vi "createSection.vi"(8 "error in (no error)":errorcluster, 10 "Style":refnum<class "Style.lvclass">, 11 "Paragraph in":refnum<k24>) -> (0 "error out":errorcluster, 2 "Section out":refnum<k24>, 3 "Paragraph out":refnum<k24>)   [LabVIEW 2017, in "LabVIEW NPOI.lvlib" / "xwpfWriter.lvclass"]
uses:
  xwpfWriter.lvclass
  Styles/Style/Style.lvclass
  C:/Users/Neo/Desktop/Dev_Tools_BR/LabVIEW_NPOI/lib/NPOI 2.1.1/NPOI.OOXML.dll
  lib/NPOI 2.1.1/NPOI.OOXML.dll
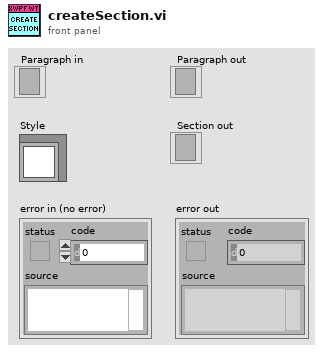
[diagram p1: front panel]
types:
  T1 = typedef "Styles.lvlib/Alignment--ring.ctl" = i32
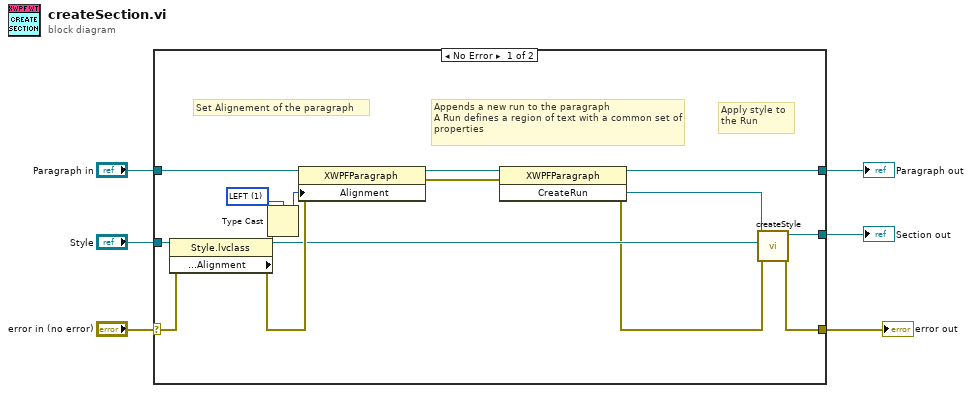
[diagram p0: block diagram]
diagram:
  n1 = case shown="No Error" "error in (no error)" {
    selector: "error in (no error)" -> [w17 w23]
    tunnel: [w12 w23] -> w5
    tunnel: "Style" -> [w21 _]
    tunnel: "Paragraph in" -> [w16 w22]
    tunnel: [w11 w22] -> w2
    tunnel: [w10 _] -> w1
    frame No Error {
      w9 = 1 items=["LEFT"=1, "CENTER"=2, "RIGHT"=3, "BOTH"=4, "MEDIUM_KASHIDA"=5, "DISTRIBUTE"=6, "NUM_TAB"=7, "HIGH_KASHIDA"=8, "LOW_KASHIDA"=9, "THAI_DISTRIBUTE"=10] ("Alignment")
      # "Apply style to\nthe Run"
      # "Set Alignement of the paragraph"
      # "Appends a new run to the paragraph\nA Run defines a region of text with a common set of properties"
      n2 = property class="Style.lvclass"(reference=w21, error in=w17) -> (reference out=w14:refnum<class "Style.lvclass">, error out=w18:errorcluster, "Public VIs:Properties:Alignment"=w8:T1)
      n3 = Type Cast(type=w9, x=w8) -> (*(type *) &x=w7:i32)
      n4 = property class="XWPFParagraph"(reference=w16, error in=w18, "Alignment"=w7) -> (reference out=w20:refnum<k24>, error out=w19:errorcluster)
      n5 = invoke class="XWPFParagraph" method="CreateRun"(reference=w20, error in=w19) -> (reference out=w11:refnum<k24>, error out=w13:errorcluster, "CreateRun"=w15:refnum<k24>)  [unwired: 1 in]
      n6 = call "createStyle.vi"("error in (no error)"=w13, "Style"=w14, "Section in"=w15) -> ("error out"=w12:errorcluster, "Section out"=w10:refnum<k24>)  [unwired: 7 in]
    }
    frame Error {
    }
  }
  "error out" <- w5
  "Paragraph out" <- w2
  "Section out" <- w1
